vi "IMAQ FPGA CoaXPress Acquisition.vi"   [LabVIEW 2020]
doc: "Acquires images from a CoaXPress camera. The VI converts the pixels from NI_AXI4-S format to a Vision Pixel Bus. The <B>Vision Pixel Bus Out</B> can be connected to Vision FPGA algorithms for processing or transferred to the host. Ensure that this VI is called from a Single Cycle Timed Loop. Use multiple instances of this VI along with <B>Device ID</B> and <B>Stream ID</B> inputs to output a Vision Pixel Bus for multiple cameras."
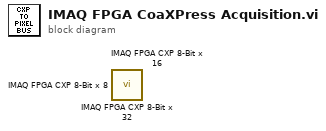
[diagram p0: block diagram]
diagram:
  n1 = call <vilib>:"IMAQ FPGA CXP 8-Bit x 32.vi"() -> ()  [unwired: 8 in, 4 out]
  n2 = call <vilib>:"IMAQ FPGA CXP 8-Bit x 16.vi"() -> ()  [unwired: 8 in, 4 out]
  n3 = call <vilib>:"IMAQ FPGA CXP 8-Bit x 8.vi"() -> ()  [unwired: 8 in, 4 out]
